vi "5_Convert 3 bit binary number into decimal.vi"() -> ()   [LabVIEW 2018]
panel:
  out "VALUE":i16
  in  "Boolean 3":bool
  in  "Boolean 2":bool
  in  "Boolean":bool
  in  "Numeric 3":dbl
  in  "Numeric 2":dbl
  in  "Numeric":dbl
  out "DECIMAL NUMBER":dbl
  in  "Button 3":bool
  in  "Button 2":bool
  in  "Button 1":bool
  # "WAP to convert 3 bit binary number into decimal"
  # "METHOD 1"
  # "METHOD 2"
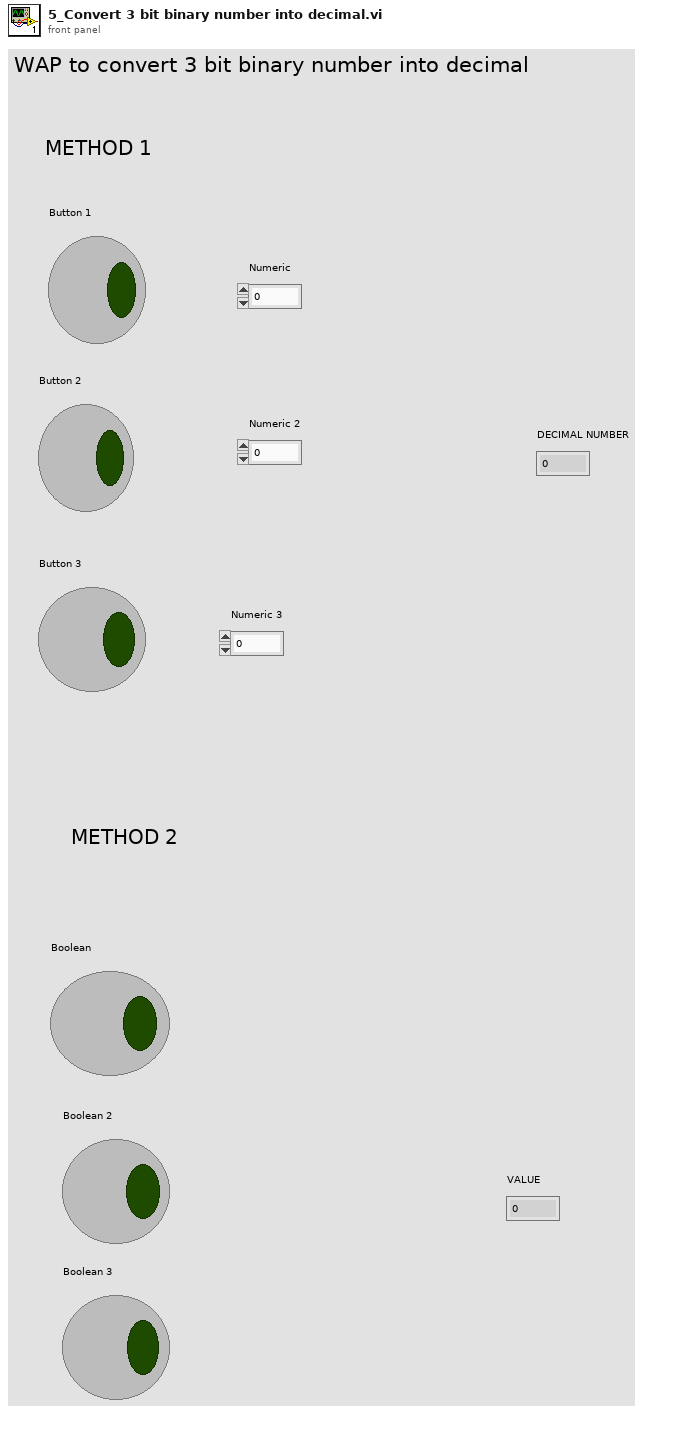
[diagram p1: front panel]
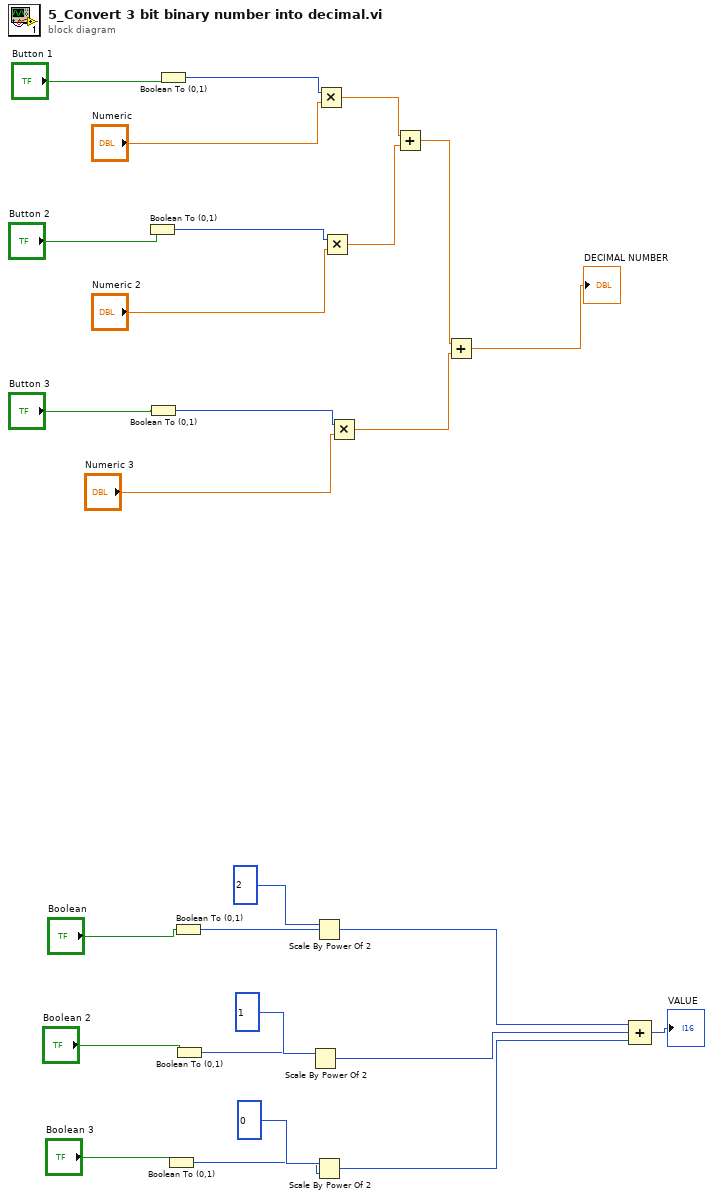
[diagram p0: block diagram]
diagram:
  n1 = Boolean To (0,1)(Boolean="Button 2") -> (0, 1=w17:i16)
  n2 = Boolean To (0,1)(Boolean="Button 3") -> (0, 1=w14:i16)
  n3 = Boolean To (0,1)(Boolean="Button 1") -> (0, 1=w25:i16)
  n4 = Boolean To (0,1)(Boolean="Boolean 3") -> (0, 1=w5:i16)
  n5 = Boolean To (0,1)(Boolean="Boolean") -> (0, 1=w7:i16)
  n6 = Boolean To (0,1)(Boolean="Boolean 2") -> (0, 1=w6:i16)
  n7 = Scale By Power Of 2(n=i16 1, x=w6) -> (x*2^n=w3:i16)
  n8 = Scale By Power Of 2(n=i16 2, x=w7) -> (x*2^n=w4:i16)
  n9 = Scale By Power Of 2(n=i16 0, x=w5) -> (x*2^n=w2:i16)
  n10 = Multiply(x=w25, y="Numeric") -> (x*y=w23:dbl)
  n11 = Multiply(x=w17, y="Numeric 2") -> (x*y=w24:dbl)
  n12 = Multiply(x=w14, y="Numeric 3") -> (x*y=w21:dbl)
  n13 = Add(x=w23, y=w24) -> (x+y=w22:dbl)
  n14 = Add(x=w22, y=w21) -> (x+y=→"DECIMAL NUMBER":dbl)
  n15 = Compound Arithmetic op=ADD(w4, w3, w2) -> (→"VALUE":i16)
